vi "only_canon.vi"(10 "열거형":enum16{"당기기", "밀기"}(ring)) -> ()   [LabVIEW 2019]
uses:
  <vilib>/Platform/TimedLoop/XDataNode/timing_clust.ctl
  <vilib>/Platform/TimedLoop/XDataNode/nitl_modes.ctl
  <vilib>/Platform/TimedLoop/XDataNode/wakeup.ctl
  <vilib>/FPGAPlugInAG/myRIO-1900/niLvFpga_Open_myRIO-1900.vi
  <vilib>/rvi/interface/common/dynamic/niFpgaDynamicAddResources.vi
  <vilib>/Utility/error.llb/Error Cluster From Error Code.vi
  <vilib>/rvi/errors/niLvFpgaAdjustHostInterfaceError.vi
  <vilib>/FPGAPlugInAG/Dynamic/niLvFpga_Close_Dynamic.vi
  <vilib>/Platform/TimedLoop/XDataNode/XDataNode.xnode
  <vilib>/rvi/interface/nirviOpenFPGA/nirviOpenFPGA.xnode
  FPGA Bitfiles/capstone_FPGATarget_encoderFPGA_AeXAVEDpCcY.lvbitx
  encoder_FPGA.vi
  <vilib>/rvi/interface/nirviReadWriteControl/nirviReadWriteControl.xnode
  <vilib>/rvi/interface/nirviCloseFPGA/nirviCloseFPGA.xnode
  <vilib>/Platform/TimedLoop/XDataNode/XDNodeRunTimeDep.lvlib
  <vilib>/rvi/interface/Simulation/niFpgaSimulationCallBeginRW.vi
  NiFpgaLv.dll
panel:
  in  "motor_stop":bool
  out "s? t:f":u32
  in  "reset":bool
  in  "정지":bool
  out "x > y?":bool
  out "타임아웃":i32
  # "F가 당기는 겅가"
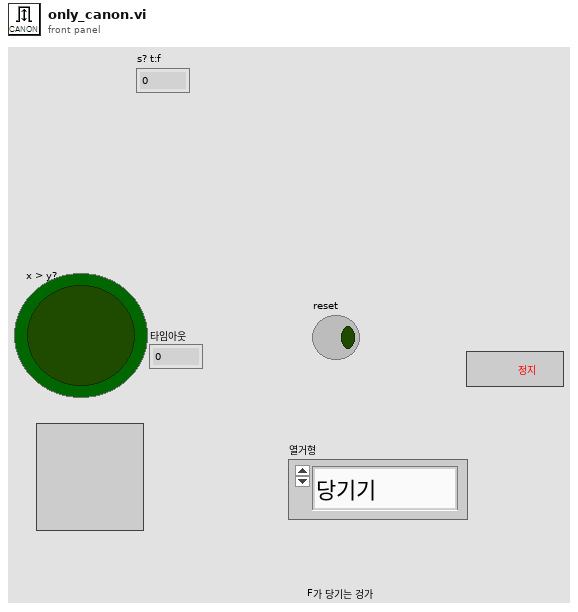
[diagram p1: front panel]
types:
  T1 = typedef "XDNodeRunTimeDep.lvlib/timing_clust.ctl" = cluster{"Expected End [f-1]":u64, "Actual End [f-1]":u64, "Finished Late? [f-1]":bool, "Expected End [i-1]":u64, "Actual End [i-1]":u64, "Finished Late? [i-1]":bool, "Expected Start [i]":u64, "Actual Start [i]":u64, "Expected Start [f]":u64, "Actual Start [f]":u64, "Source Name":string, "Structure Name":string, "Period":i64, "Deadline":i64, "Offset":i64, "Start":i64, "Priority":i32, "Timeout":i32, "Mode":T2, "Wakeup Reason":T3, "Error":errorcluster, "Source Type":string, "Secondary Source Type":string, "Global End Time":u64, "Global Start Time":u64, "Frame Duration":u64, "Iteration Duration":u64, "Assigned CPU":i32, "I/O Scan Engine Mode":u32}
  T2 = typedef "XDNodeRunTimeDep.lvlib/nitl_modes.ctl" = enum32{"No Change", "Process missed periods, maintain original phase", "Discard missed periods, maintain original phase", "Process missed periods, ignore original phase", "Discard missed periods, ignore original phase"}
  T3 = typedef "XDNodeRunTimeDep.lvlib/wakeup.ctl" = enum32{"Normal", "Aborted", "Asynchronous wakeup", "Timing source error", "Timed loop error", "Timeout"}
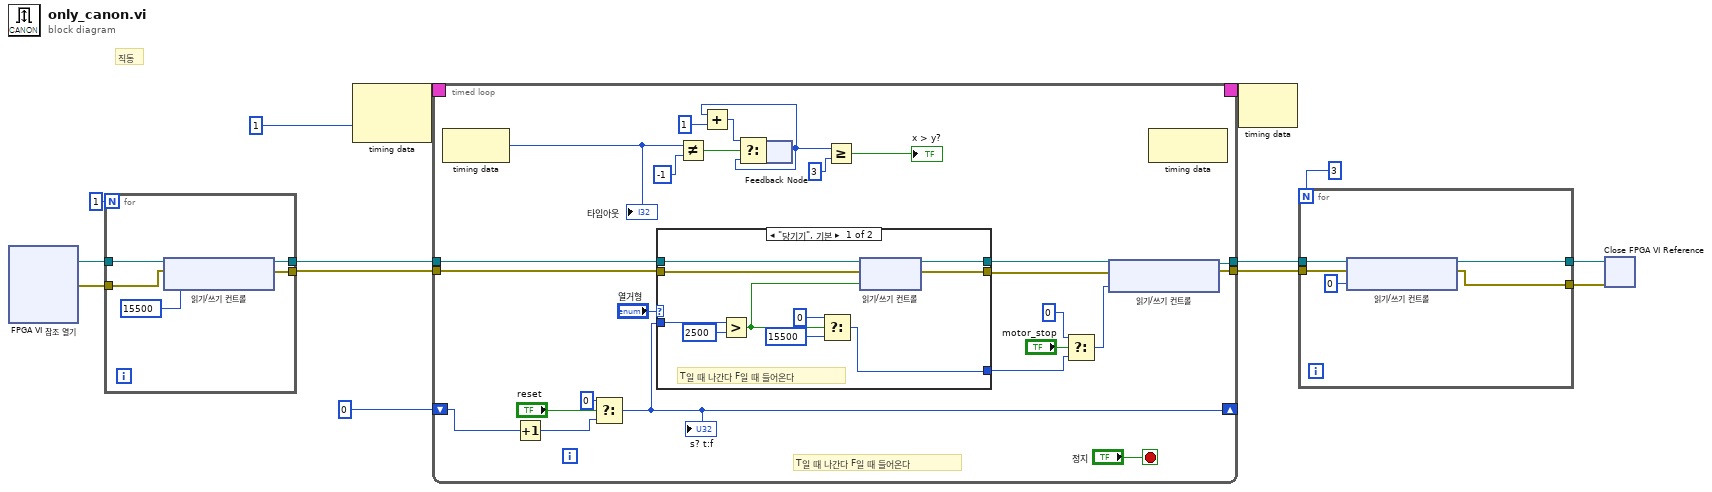
[diagram p0: block diagram]
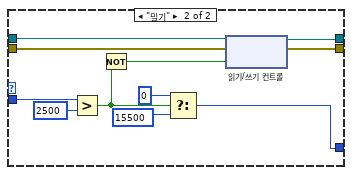
[diagram p2: hidden frame]
diagram:
  # "직동"
  n1 = xnode "FPGA VI 참조 열기"() -> ("FPGA VI 참조 출력"=w5:refnum<k20>, "에러 출력"=w4:errorcluster)  [unwired: 2 in]
  n2 = for {
    N: 1 -> [_]
    tunnel: [w19] -> w7
    tunnel: [w18] -> w6
    tunnel: w5 -> [w16]
    tunnel: w4 -> [w15]
    n3 = xnode "읽기/쓰기 컨트롤"("FPGA VI 참조 입력"=w16, "에러 입력"=w15, "직동_pwm input"=15500) -> ("FPGA VI 참조 출력"=w19:refnum<k20>, "에러 출력"=w18:errorcluster)
  }
  n4 = node-c288(i64 1 ("주기")) -> (w14:T1)  [unwired: 1 in]
  n5 = timed-loop {
    timing: w14 -> [_]
    timing-out: [_] -> w13
    tunnel: w7 -> [w35]
    tunnel: w6 -> [w34]
    tunnel: [w25] -> w12
    tunnel: [w24] -> w11
    shift-right: [w28] -> _
    shift-left: u32 0 ("y") -> [w30]
    stop <- "정지" stop-if-true
    # "T일 때 나간다 F일 때 들어온다"
    n6 = node-c288() -> (w45:i32)  [unwired: 1 in]
    "타임아웃" <- w45
    n7 = Increment(x=w30) -> (x+1=w29:u32)
    n8 = Select(t=u32 0, s="reset", f=w29) -> (s? t:f=w28:u32)
    "s? t:f" <- w28
    n9 = case shown="\"당기기\", 기본" "열거형" {
      tunnel: w35 -> [w54 w64]
      tunnel: w34 -> [w53 w61]
      tunnel: [w52 w63] -> w27
      tunnel: [w51 w62] -> w26
      tunnel: w28 -> [w50 w60]
      tunnel: [w46 w56] -> w22
      frame "당기기", Default {
        # "T일 때 나간다 F일 때 들어온다"
        n10 = Greater?(x=w50, y=2500) -> (0:w47:bool)
        n11 = Select(t=0, s=w47, f=15500) -> (s? t:f=w46:i32)
        n12 = xnode "읽기/쓰기 컨트롤"("FPGA VI 참조 입력"=w54, "에러 입력"=w53, "직동_dir"=w47) -> ("FPGA VI 참조 출력"=w52:refnum<k20>, "에러 출력"=w51:errorcluster)
      }
      frame "밀기" {
        n13 = Greater?(x=w60, y=2500) -> (0:w59:bool)
        n14 = Not(x=w59) -> (.not. x?=w65:bool)
        n15 = Select(t=0, s=w59, f=15500) -> (s? t:f=w56:i32)
        n16 = xnode "읽기/쓰기 컨트롤"("FPGA VI 참조 입력"=w64, "에러 입력"=w61, "직동_dir"=w65) -> ("FPGA VI 참조 출력"=w63:refnum<k20>, "에러 출력"=w62:errorcluster)
      }
    }
    n17 = Not Equal?(x=w45, y=-1) -> (x != y?=w43:bool)
    n18 = feedback #1() -> (w39:u8)  [unwired: 1 in]
    n19 = Add(x=w39, y=u8 1) -> (x+y=w42:u8)
    n20 = Select(t=w42, s=w43, f=w39) -> (s? t:f=w41:u8)
    n21 = feedback-in #1(w41) -> ()
    n22 = Greater Or Equal?(x=w39, y=u8 3) -> (x >= y?=→"x > y?":bool)
    n23 = Select(t=0, s="motor_stop", f=w22) -> (s? t:f=w20:i32)
    n24 = xnode "읽기/쓰기 컨트롤"("FPGA VI 참조 입력"=w27, "에러 입력"=w26, "직동_pwm input"=w20) -> ("FPGA VI 참조 출력"=w25:refnum<k20>, "에러 출력"=w24:errorcluster)
    n25 = node-c288() -> ()  [unwired: 1 in, 1 out]
  }
  n26 = node-c288(w13) -> ()  [unwired: 1 out]
  n27 = for {
    N: 3 -> [_]
    tunnel: w12 -> [w74]
    tunnel: w11 -> [w73]
    tunnel: [w71] -> w3
    tunnel: [w70] -> w2
    n28 = xnode "읽기/쓰기 컨트롤"("FPGA VI 참조 입력"=w74, "에러 입력"=w73, "직동_pwm input"=0) -> ("FPGA VI 참조 출력"=w71:refnum<k20>, "에러 출력"=w70:errorcluster)
  }
  n29 = xnode "Close FPGA VI Reference"("FPGA VI 참조 입력"=w3, "에러 입력"=w2) -> ()  [unwired: 1 out]
